vi "Convert to Outcome.vi"(9 "Error":errorcluster, 10 "Is Assertion?":bool, 11 "Pass?":bool) -> (3 "Outcome":T1=enum."Skipped")   [LabVIEW 2020, in "MacroAssert.lvlib"]
uses:
  MacroAssert.lvlib
  CTLs/Outcome.ctl
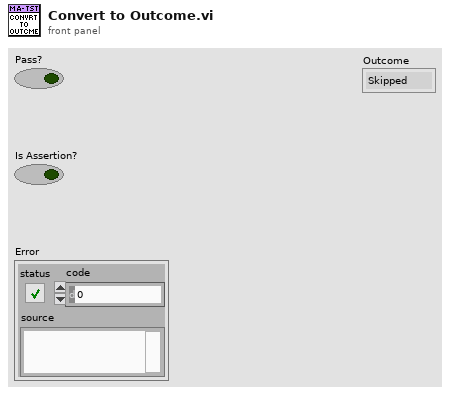
[diagram p1: front panel]
types:
  T1 = typedef "MacroAssert.lvlib/Outcome.ctl" = enum16{"Not Started", "Skipped", "Pass", "Fail", "Complete", "Error", "Auto Abort", "User Abort"}
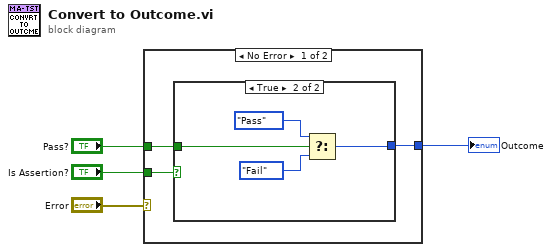
[diagram p0: block diagram]
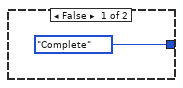
[diagram p2: hidden frame]
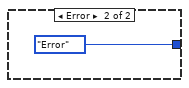
[diagram p3: hidden frame]
diagram:
  n1 = case shown="No Error" "Error" {
    tunnel: "Pass?" -> [w7 _]
    tunnel: [w5 Outcome."Error" ("Result")] -> w2
    tunnel: "Is Assertion?" -> [w6 _]
    frame No Error {
      n2 = case shown="True" w6 {
        tunnel: w7 -> [_ w12]
        tunnel: [Outcome."Complete" ("Result") w9] -> w5
        frame False {
        }
        frame True {
          n3 = Select(t=Outcome."Pass" ("Result"), s=w12, f=Outcome."Fail" ("Result")) -> (s? t:f=w9:T1)
        }
      }
    }
    frame Error {
    }
  }
  "Outcome" <- w2
